vi "Read I16.vi"(11 "Event in":refnum<class "Event I16.lvclass">) -> (2 "I16":i16, 3 "Event out":refnum<class "Event I16.lvclass">)   [LabVIEW 2016, in "Event Source.lvlib" / "Event I16.lvclass"]
uses:
  Event I16.lvclass
  Event I16.lvclass/Event I16.ctl
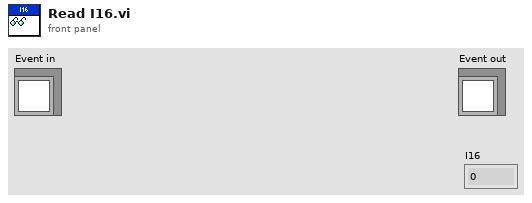
[diagram p1: front panel]
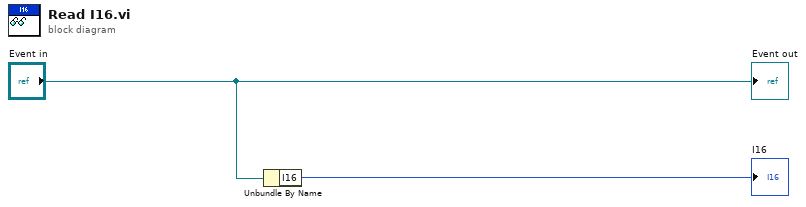
[diagram p0: block diagram]
diagram:
  n1 = Unbundle By Name("Event in") -> ("I16"=→"I16":i16)
  "Event out" <- "Event in"
